vi "InitTileBufferFromFile.vi"(8 "error in (no error)":errorcluster, 10 "Tile Path":path, 11 "Refnum in":T1) -> (0 "error out":errorcluster, 3 "Refnum out":T1)   [LabVIEW 2019, in "RT_Game.lvlib" / "Engine.lvclass"]
uses:
  Engine.lvclass
  FPGA_Interface.ctl
  <vilib>/rvi/interface/common/niFpgaWaitOnOcc.vi
  <vilib>/Utility/error.llb/Error Cluster From Error Code.vi
  <vilib>/rvi/errors/niLvFpgaAdjustHostInterfaceError.vi
  <vilib>/rvi/interface/nirviMethod/nirviMethod.xnode
  FPGA Bitfiles/myriogameconsole_FPGATarget_Main_ntsPRcBZGxk.lvbitx
  <vilib>/rvi/interface/nirviReadWriteControl/nirviReadWriteControl.xnode
  <vilib>/rvi/errors/niLvFpgaMergeErrorWithErrorCode.vi
  NiFpgaLv.dll
  <vilib>/FPGAPlugInAG/myRIO-1900/niLvFpga_ConfigureFifo_myRIO-1900.vi
  <vilib>/FPGAPlugInAG/myRIO-1900/niLvFpga_WriteFifo_myRIO-1900.vi
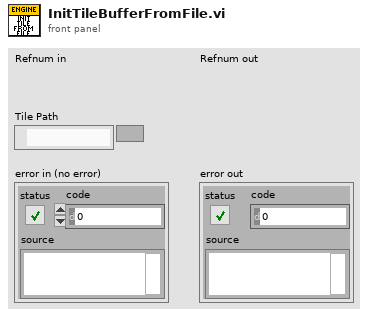
[diagram p1: front panel]
types:
  T1 = typedef "FPGA_Interface.ctl" = refnum<k20>
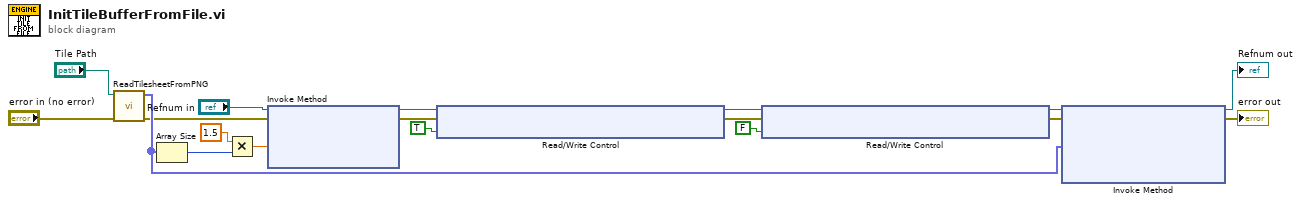
[diagram p0: block diagram]
diagram:
  n1 = call "ReadTilesheetFromPNG.vi"("error in (no error)"="error in (no error)", "path to PNG file"="Tile Path") -> ("error out"=w4:errorcluster, "TileBufferData"=w15:fxp<+,3,3>[])  [unwired: 8 in]
  n2 = Array Size(array=w15) -> (size(s)=w16:i32)
  n3 = Multiply(x=1.5, y=w16) -> (x*y=w17:dbl)
  n4 = xnode "Invoke Method"("FPGA VI Reference In"="Refnum in", "error in"=w4, "Requested Depth"=w17) -> ("FPGA VI Reference Out"=w14:T1, "error out"=w12:errorcluster)  [unwired: 1 out]
  n5 = xnode "Read/Write Control"("FPGA VI Reference In"=w14, "error in"=w12, "Tilesetbuffer_ResetAddress"=TRUE ("Tilebuffer_ResetAddress")) -> ("FPGA VI Reference Out"=w10:T1, "error out"=w9:errorcluster)
  n6 = xnode "Read/Write Control"("FPGA VI Reference In"=w10, "error in"=w9, "Tilesetbuffer_ResetAddress"=FALSE ("Tilebuffer_ResetAddress")) -> ("FPGA VI Reference Out"=w8:T1, "error out"=w7:errorcluster)
  n7 = xnode "Invoke Method"("FPGA VI Reference In"=w8, "error in"=w7, "Data"=w15) -> ("FPGA VI Reference Out"=→"Refnum out":T1, "error out"=→"error out":errorcluster)  [unwired: 1 in, 1 out]
